vi "smooth 2D - x then y.vi"(11 "2D array":dbl[][](array[numeric])=array200x300[60000 elements]) -> (0 "x+y":dbl[][](array[numeric]))   [LabVIEW 2014]
uses:
  <vilib>/Analysis/3filter.llb/Zero Phase Filter (DBL).vi
  <vilib>/Analysis/NI_AALBase.lvlib
panel:
  in  "shape 3":enum16{"rectangular", "triangular"}(ring)
  in  "half-width 3":i32=8
  in  "type 3":enum16{"moving average", "exponential"}(ring)
  in  "time constant 3":dbl=0.1 format="%.2f"
  in  "fs 3":dbl=0.01 format="%0.2f"
  in  "shape 2":enum16{"rectangular", "triangular"}(ring)
  in  "half-width 2":i32=8
  in  "type 2":enum16{"moving average", "exponential"}(ring)
  in  "time constant 2":dbl=0.1 format="%.2f"
  in  "fs 2":dbl=0.01 format="%0.2f"
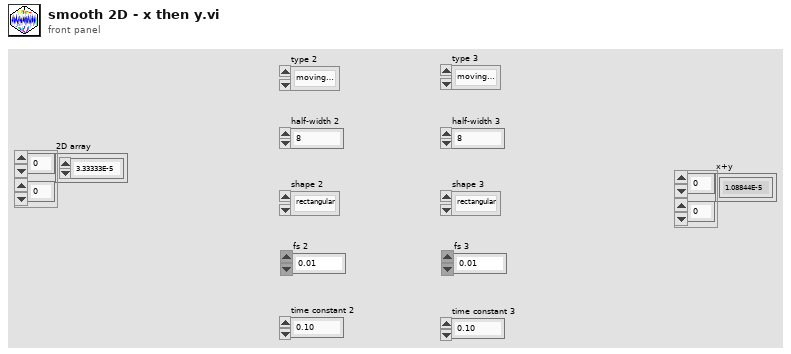
[diagram p1: front panel]
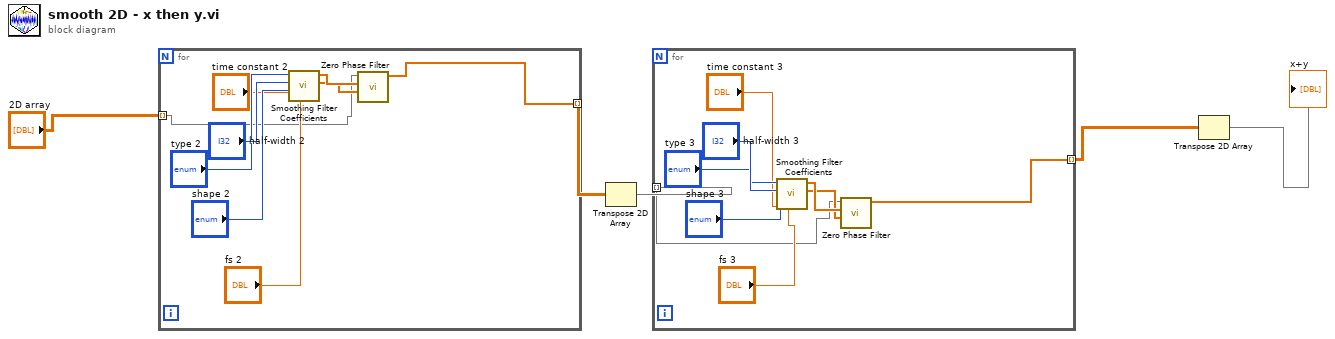
[diagram p0: block diagram]
diagram:
  n1 = for {
    tunnel: [w11] -> w3 mode=indexing
    tunnel: "2D array" -> [w6] mode=indexing
    n2 = call <vilib>:"Smoothing Filter Coefficients.vi"("fs"="fs 2", "time constant"="time constant 2", "shape"="shape 2", "half-width"="half-width 2", "type"="type 2") -> ("forward coefficients"=w7:dbl[], "reverse coefficients"=w8:dbl[])  [unwired: 4 in, 1 out]
    n3 = call-poly <vilib>:"Zero Phase Filter.vi"("Forward Coefficients"=w7, "Reverse Coefficients"=w8, "X"=w6) -> ("Filtered X"=w11:dbl[])  [unwired: 7 in, 1 out]
  }
  n4 = Transpose 2D Array(2D array=w3) -> (transposed array=w5:dbl[][])
  n5 = for {
    tunnel: w5 -> [w15] mode=indexing
    tunnel: [w20] -> w1 mode=indexing
    n6 = call <vilib>:"Smoothing Filter Coefficients.vi"("fs"="fs 3", "time constant"="time constant 3", "shape"="shape 3", "half-width"="half-width 3", "type"="type 3") -> ("forward coefficients"=w16:dbl[], "reverse coefficients"=w17:dbl[])  [unwired: 4 in, 1 out]
    n7 = call-poly <vilib>:"Zero Phase Filter.vi"("Forward Coefficients"=w16, "Reverse Coefficients"=w17, "X"=w15) -> ("Filtered X"=w20:dbl[])  [unwired: 7 in, 1 out]
  }
  n8 = Transpose 2D Array(2D array=w1) -> (transposed array=→"x+y":dbl[][])
